vi "U3 Create All Message Queues.vi"(8 "error in (no error)":errorcluster, 11 "Process Name":string) -> (0 "error out":errorcluster, 3 "Message Queues":T1)   [LabVIEW 2018, in "U3 Module.lvlib"]
uses:
  Pump Module Folder/All Message Queues.ctl
  support/Message Queue/Message Cluster.ctl
  Config Module/Controls/OP Window Display.ctl
  Pump Module Folder/Pump Module Display.ctl
  support/Message Queue/Enqueue Message (Single).vi
  U3 Module.lvlib
  support/Message Queue/Message Queue.lvlib
  Pump Module Folder/Pump Module.lvlib
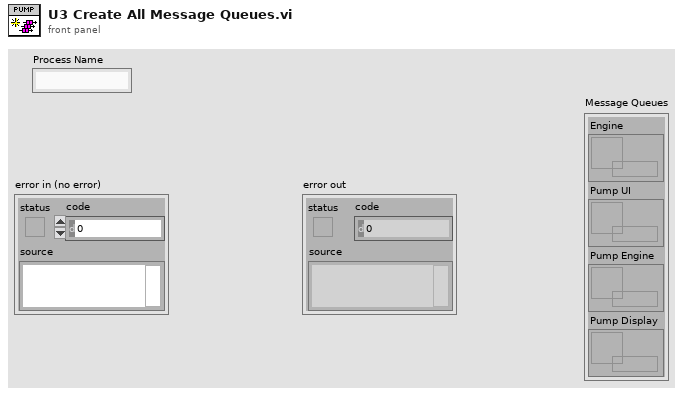
[diagram p1: front panel]
types:
  T1 = typedef "Pump Module.lvlib/All Message Queues.ctl" = cluster{"Engine":refnum<queue>, "Pump UI":refnum<queue>, "Pump Engine":refnum<queue>, "Pump Display":refnum<queue>}
  T2 = typedef "Pump Module.lvlib/Pump Module Display.ctl" = cluster{"Pump On?":bool, "Cycle Period":dbl, "Current Pump Speed":dbl}
  T3 = typedef "OP Window Display.ctl" = cluster{"Flow":dbl, "PID2 Out":dbl}
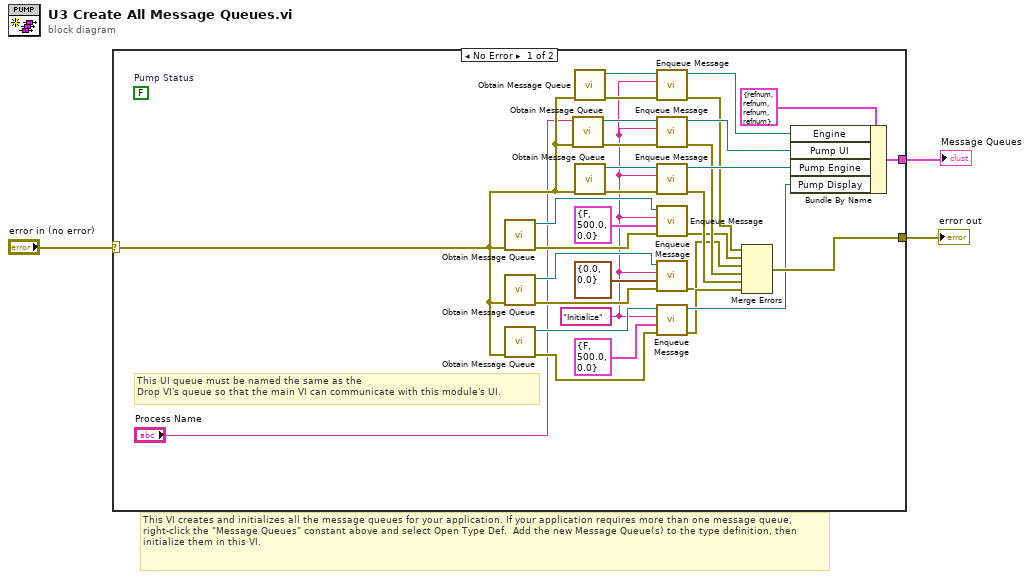
[diagram p0: block diagram]
diagram:
  # "This VI creates and initializes all the message queues for your application. If your application requires more than one message queue, right-click the \"Message Queues\" constant above and select Open Type Def.  Add the new Message Queue(s) to the type definition, then initialize them in this VI."
  n1 = case shown="No Error" "error in (no error)" {
    selector: "error in (no error)" -> [w12 w35]
    tunnel: [w33 w35] -> w3
    tunnel: [w34 _] -> w1
    frame No Error {
      (unwired) FALSE  # Pump Status
      w4 = "Initialize" ("Message")
      # "This UI queue must be named the same as the \nDrop VI's queue so that the main VI can communicate with this module's UI."
      n2 = call "Obtain Message Queue.vi"("error in (no error)"=w12) -> ("error out"=w29:errorcluster, "Message Queue"=w28:refnum<queue>)  [unwired: 9 in]
      n3 = call "Obtain Message Queue.vi"("error in (no error)"=w12) -> ("error out"=w27:errorcluster, "Message Queue"=w26:refnum<queue>)  [unwired: 9 in]
      n4 = call "Obtain Message Queue.vi"("error in (no error)"=w12) -> ("error out"=w20:errorcluster, "Message Queue"=w21:refnum<queue>)  [unwired: 9 in]
      n5 = call "Obtain Message Queue.vi"("error in (no error)"=w12, "name (unnamed)"="Process Name") -> ("error out"=w13:errorcluster, "Message Queue"=w24:refnum<queue>)  [unwired: 8 in]
      n6 = call "Obtain Message Queue.vi"("error in (no error)"=w12) -> ("error out"=w31:errorcluster, "Message Queue"=w32:refnum<queue>)  [unwired: 9 in]
      n7 = call "Obtain Message Queue.vi"("error in (no error)"=w12) -> ("error out"=w22:errorcluster, "Message Queue"=w23:refnum<queue>)  [unwired: 9 in]
      n8 = call-poly "Enqueue Message.vi"("error in (no error)"=w31, "Message"=w4, "Message Queue"=w32) -> ("error out"=w5:errorcluster, "dup Message Queue"=w30:refnum<queue>)  [unwired: 7 in]
      n9 = call-poly "Enqueue Message.vi"("error in (no error)"=w13, "Message"=w4, "Message Queue"=w24) -> ("error out"=w16:errorcluster, "dup Message Queue"=w19:refnum<queue>)  [unwired: 7 in]
      n10 = call-poly "Enqueue Message.vi"("error in (no error)"=w22, "Message"=w4, "Message Queue"=w23) -> ("error out"=w15:errorcluster, "dup Message Queue"=w18:refnum<queue>)  [unwired: 7 in]
      n11 = call-poly "Enqueue Message.vi"("error in (no error)"=w29, "Message Data"=T2 {"Pump On?"=FALSE, "Cycle Period"=500.0, "Current Pump Speed"=0.0} ("PM Display"), "Message"=w4, "Message Queue"=w28) -> ("error out"=w6:errorcluster)  [unwired: 6 in, 1 out]
      n12 = call-poly "Enqueue Message.vi"("error in (no error)"=w27, "Message Data"=T3 {"Flow"=0.0, "PID2 Out"=0.0}, "Message"=w4, "Message Queue"=w26) -> ("error out"=w7:errorcluster)  [unwired: 6 in, 1 out]
      n13 = call-poly "Enqueue Message.vi"("error in (no error)"=w20, "Message Data"=T2 {"Pump On?"=FALSE, "Cycle Period"=500.0, "Current Pump Speed"=0.0} ("FM Display"), "Message"=w4, "Message Queue"=w21) -> ("error out"=w14:errorcluster, "dup Message Queue"=w17:refnum<queue>)  [unwired: 6 in]
      n14 = Merge Errors(w5, w6, w7, w16, w15, w14) -> (w33:errorcluster)
      n15 = Bundle By Name(cluster=T1 {"Engine"=refnum, "Pump UI"=refnum, "Pump Engine"=refnum, "Pump Display"=refnum} ("Message Queues"), "Engine"=w30, "Pump UI"=w19, "Pump Engine"=w18, "Pump Display"=w17) -> (w34:T1)
    }
    frame Error {
    }
  }
  "Message Queues" <- w1
  "error out" <- w3
